vi "Main.vi"() -> ()   [LabVIEW 2013]
panel:
  in  "Upper Frequency Cutoff":dbl
  out "Derived Data":dbl[][](array[numeric])
  out "Processed Data":dbl[][](array[numeric])
  out "Raw Data":dbl[][](array[numeric])
  in  "Export Processed Data":bool
  in  "Process Data":bool
  in  "Time Units":enum16{"Seconds", "Minutes", "Hours"}(ring)
  in  "Data Type":enum16{"Raw", "Processed", "Derived"}(ring)
  in  "Derived Data to Display":enum16{"Altitude"}(ring)
  in  "Processed Data to Display":T1(ring)
  in  "Raw Data to Display":T1(ring)
  in  "Stop":bool
  out "error out":errorcluster
  in  "error in (no error)":errorcluster
  out "Displayed Data":cluster{dbl[], dbl[]}[](graph)
  in  "Raw Data File Path":path
  # "Processing Settings"
  # "Data Display Settings"
  # "Copyright (c) 2014 Andrew Donelick\nAll rights reserved. \n\nFor information, contact:\n<adonelick@hmc.edu>"
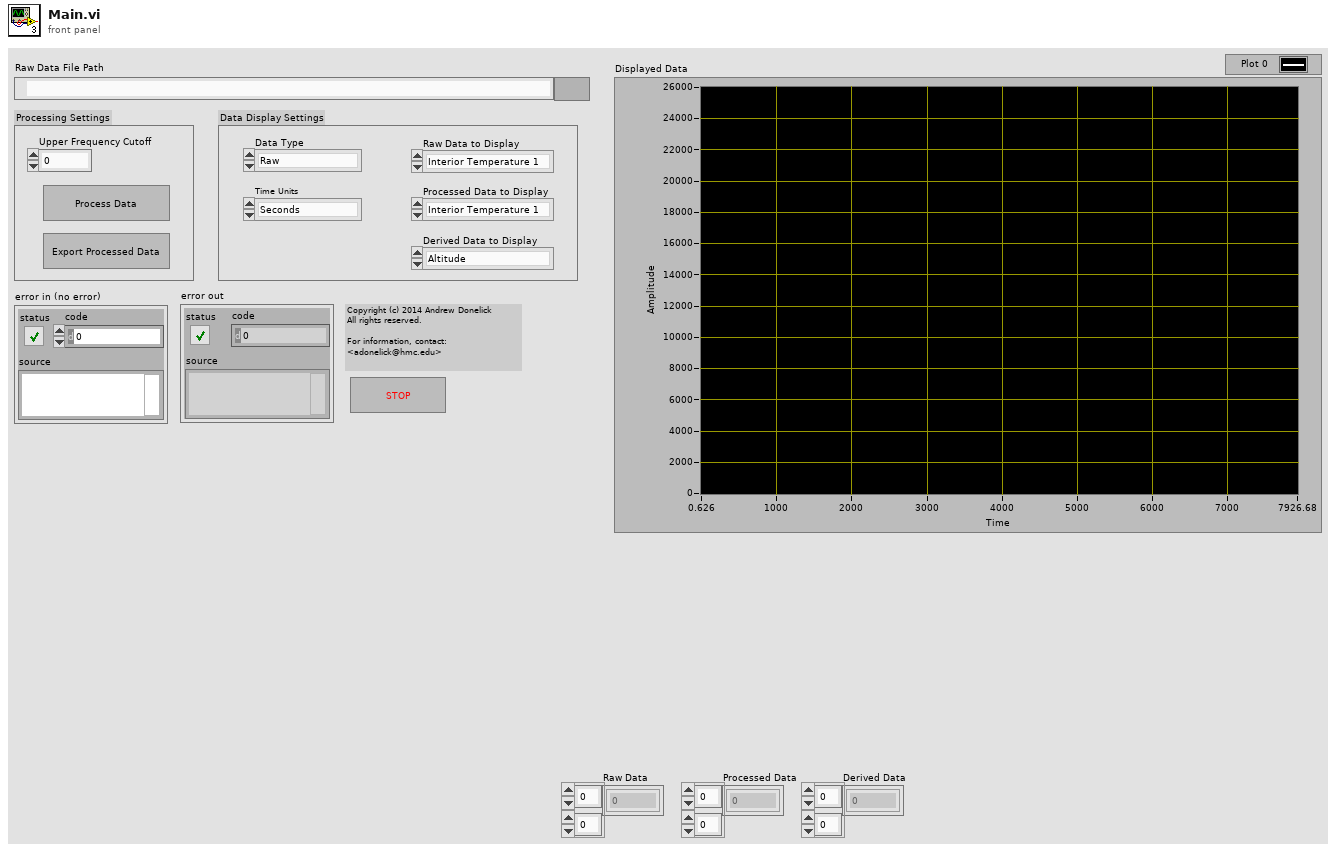
[diagram p1: front panel]
types:
  T1 = enum16{"Interior Temperature 1", "Interior Temperature 2", "Heater Temperature", "Exterior Temperature", "Humidity", "Pressure", "Pitch", "Roll", "Yaw", "Heater Status", "Relay States"}
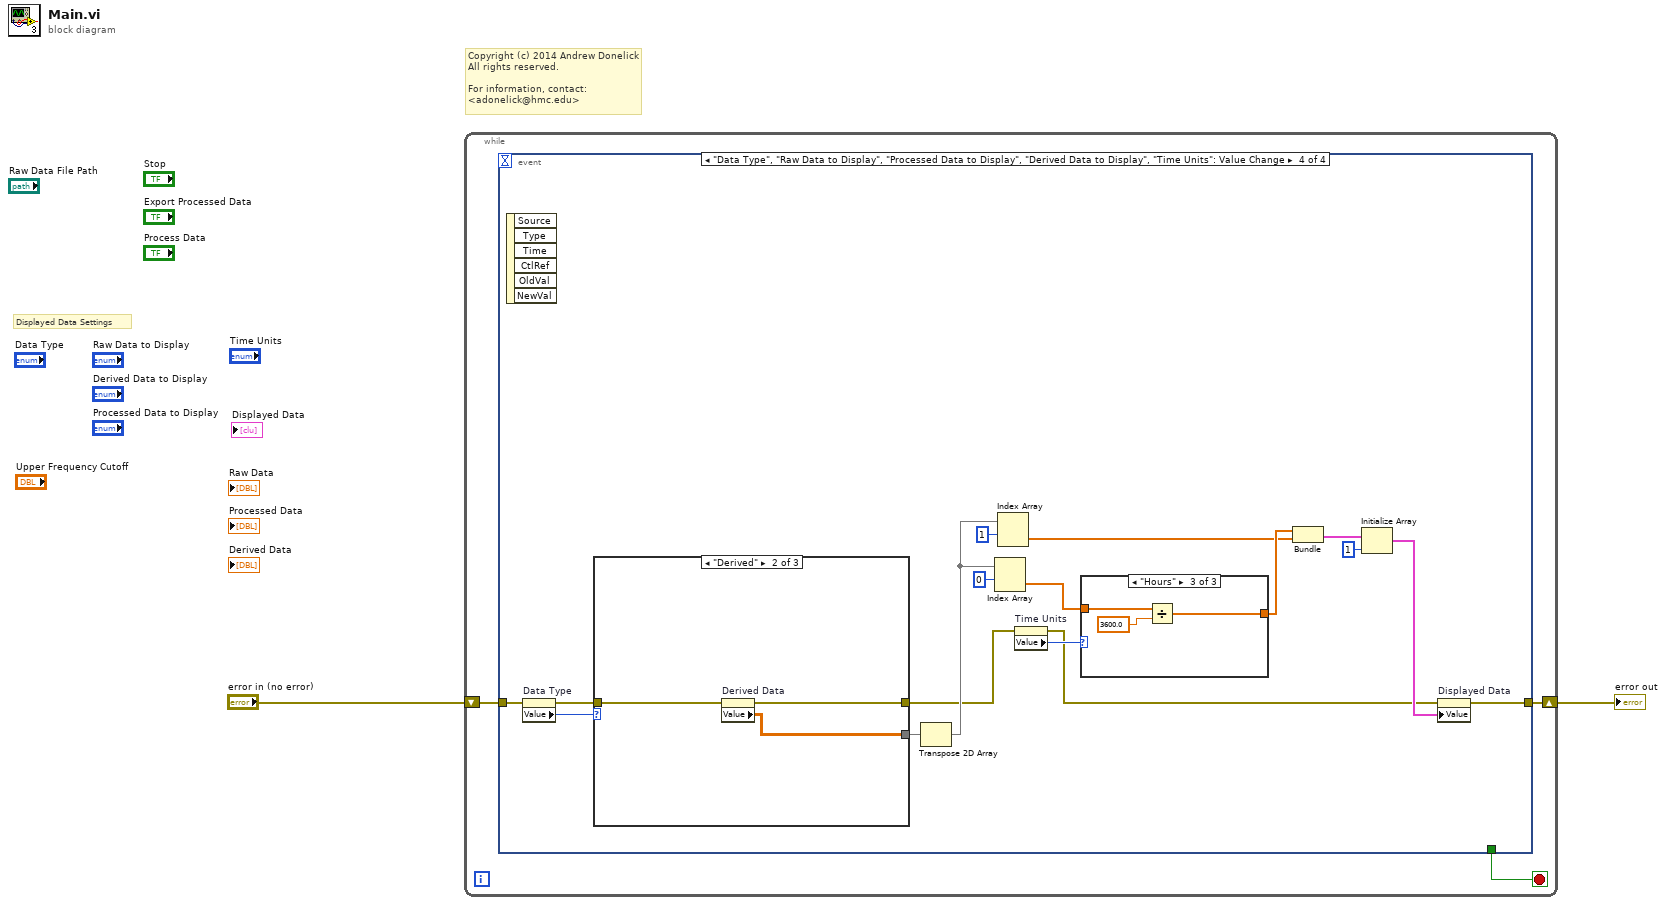
[diagram p0: block diagram]
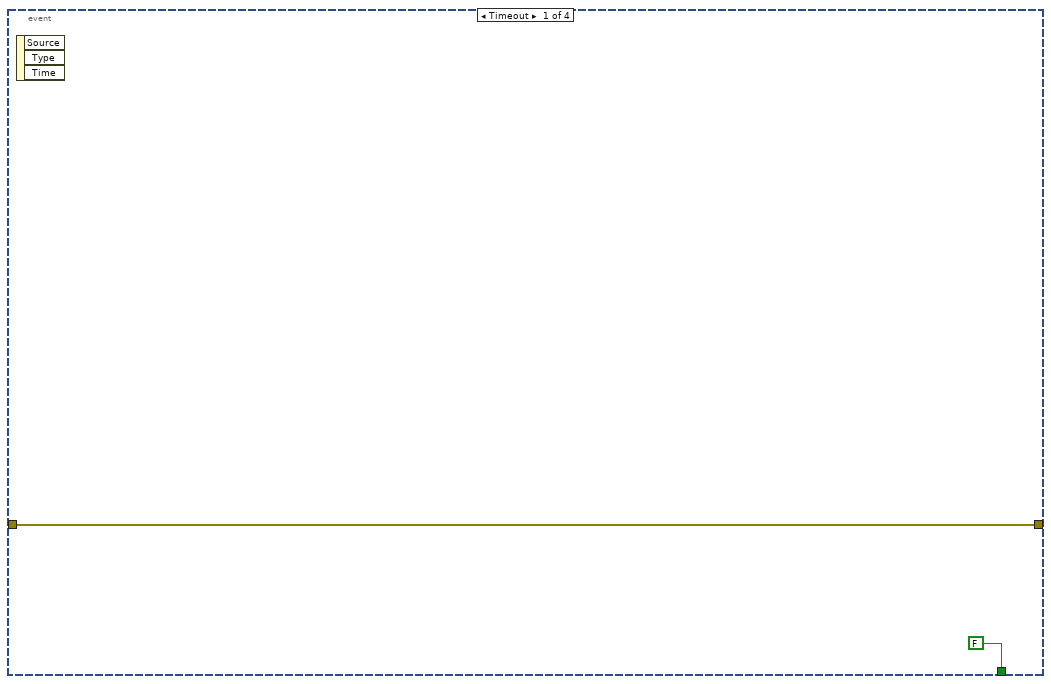
[diagram p2: hidden frame]
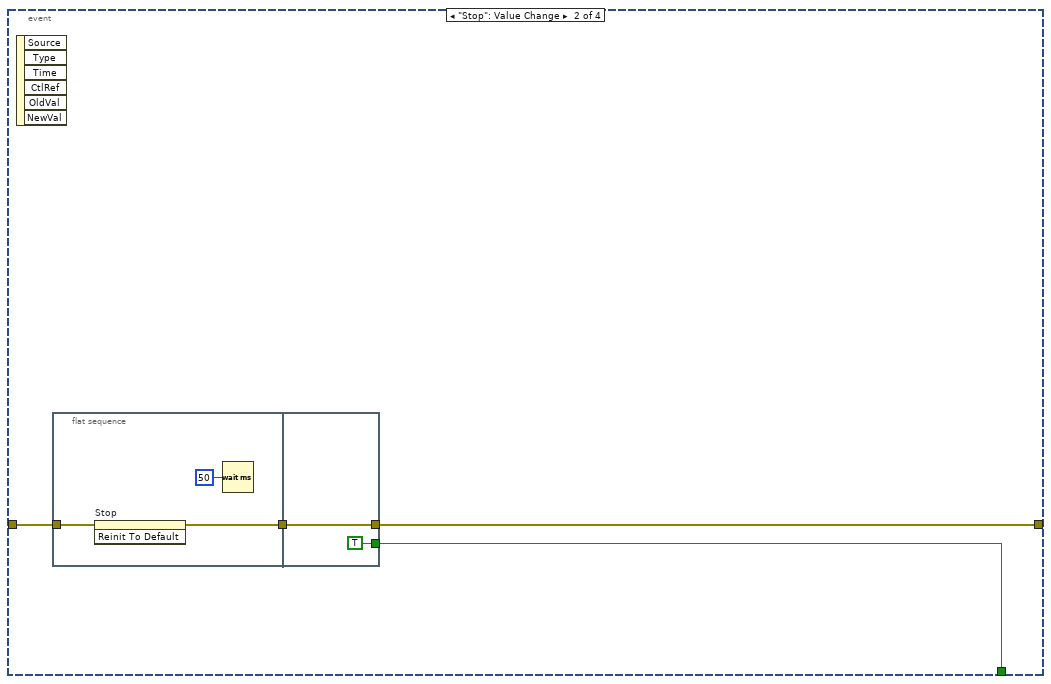
[diagram p3: hidden frame]
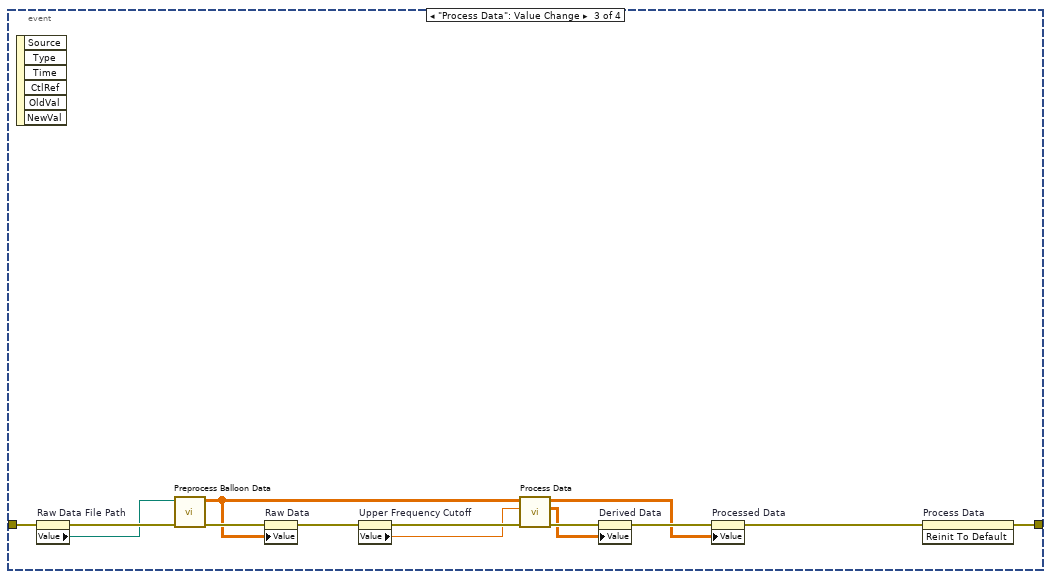
[diagram p4: hidden frame]
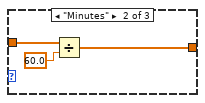
[diagram p6: hidden frame]
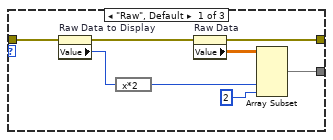
[diagram p7: hidden frame]
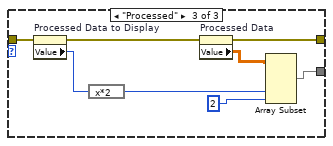
[diagram p8: hidden frame]
diagram:
  # "Copyright (c) 2014 Andrew Donelick\nAll rights reserved. \n\nFor information, contact:\n<adonelick@hmc.edu>"
  # "Displayed Data Settings"
  n1 = while {
    shift-right: [w3] -> w1
    shift-left: "error in (no error)" -> [w4]
    stop <- w5 stop-if-true
    n2 = event shown="[3] \"Data Type\", \"Raw Data to Display\", \"Processed Data to Display\", \"Derived Data to Display\", \"Time Units\": Value Change" {
      selector: _ -> [_ _ _ _]
      dyn-events: _ -> [_ _ _ _]
      timeout: _ -> [_ _ _ _]
      tunnel: [FALSE w9 _ _] -> w5
      tunnel: w4 -> [w6 w11 w29 w47]
      tunnel: [w6 w8 w30 w33] -> w3
      event Timeout {
        n3 = event-data() -> ()  [unwired: 1 in, 3 out]
      }
      event "Stop": Value Change {
        n4 = event-data() -> ()  [unwired: 1 in, 6 out]
        n5 = flat-sequence {
          tunnel: w11 -> [w14]
          tunnel: [w13] -> w10
          tunnel: w10 -> [w15]
          tunnel: [TRUE] -> w9
          tunnel: [w15] -> w8
          frame #0 {
            n6 = invoke on="Stop" class="Bool" method="Reinit To Default"(error in=w14) -> (error out=w13:errorcluster)  [unwired: 2 in, 2 out]
            n7 = Wait (ms)(milliseconds to wait=u32 50) -> ()  [unwired: 1 out]
          }
          frame #1 {
          }
        }
      }
      event "Process Data": Value Change {
        n8 = event-data() -> ()  [unwired: 1 in, 6 out]
        n9 = property on="Raw Data File Path" class="Path"(error in=w29) -> (error out=w28:errorcluster, "Value"=w27:path)  [unwired: 1 in, 1 out]
        n10 = call "Preprocess Balloon Data.vi"("error in (no error)"=w28, "Input Data File Path"=w27) -> ("error out"=w26:errorcluster, "Preprocessed Data"=w25:dbl[][])  [unwired: 8 in]
        n11 = property on="Raw Data" class="Arr (strict)"(error in=w26, "Value"=w25) -> (error out=w19:errorcluster)  [unwired: 1 in, 1 out]
        n12 = property on="Upper Frequency Cutoff" class="DigNum (strict)"(error in=w19) -> (error out=w18:errorcluster, "Value"=w17:dbl)  [unwired: 1 in, 1 out]
        n13 = call "Process Data.vi"("error in (no error)"=w18, "Upper Frequency Cutoff"=w17, "Raw Data"=w25) -> ("error out"=w24:errorcluster, "Altitude"=w22:dbl[][], "Processed Data"=w21:dbl[][])  [unwired: 6 in]
        n14 = property on="Derived Data" class="Arr (strict)"(error in=w24, "Value"=w22) -> (error out=w23:errorcluster)  [unwired: 1 in, 1 out]
        n15 = property on="Processed Data" class="Arr (strict)"(error in=w23, "Value"=w21) -> (error out=w20:errorcluster)  [unwired: 1 in, 1 out]
        n16 = invoke on="Process Data" class="Bool" method="Reinit To Default"(error in=w20) -> (error out=w30:errorcluster)  [unwired: 2 in, 2 out]
      }
      event "Data Type", "Raw Data to Display", "Processed Data to Display", "Derived Data to Display", "Time Units": Value Change {
        n17 = event-data() -> ()  [unwired: 1 in, 6 out]
        n18 = property on="Data Type" class="Enum (strict)"(error in=w47) -> (error out=w45:errorcluster, "Value"=w46:enum16{"Raw", "Processed", "Derived"})  [unwired: 1 in, 1 out]
        n19 = case shown="\"Derived\"" w46 {
          tunnel: w45 -> [w62 w65 w73]
          tunnel: [w55 w64 w72] -> w34
          tunnel: [w56 w63 w66] -> w35
          frame "Raw", Default {
            n20 = property on="Raw Data to Display" class="Enum (strict)"(error in=w62) -> (error out=w60:errorcluster, "Value"=w61:T1)  [unwired: 1 in, 1 out]
            n21 = expression code="x*2"(w61) -> (w58:T1)
            n22 = property on="Raw Data" class="Arr (strict)"(error in=w60) -> (error out=w55:errorcluster, "Value"=w59:dbl[][])  [unwired: 1 in, 1 out]
            n23 = Array Subset(array=w59, index (col)=w58, length (col)=2 ("length")) -> (w56:dbl[][])  [unwired: 2 in]
          }
          frame "Derived" {
            n24 = property on="Derived Data" class="Arr (strict)"(error in=w65) -> (error out=w64:errorcluster, "Value"=w63:dbl[][])  [unwired: 1 in, 1 out]
          }
          frame "Processed" {
            n25 = property on="Processed Data to Display" class="Enum (strict)"(error in=w73) -> (error out=w71:errorcluster, "Value"=w70:T1)  [unwired: 1 in, 1 out]
            n26 = expression code="x*2"(w70) -> (w68:T1)
            n27 = property on="Processed Data" class="Arr (strict)"(error in=w71) -> (error out=w72:errorcluster, "Value"=w69:dbl[][])  [unwired: 1 in, 1 out]
            n28 = Array Subset(array=w69, index (col)=w68, length (col)=2 ("disabled index (col)")) -> (w66:dbl[][])  [unwired: 2 in]
          }
        }
        n29 = Transpose 2D Array(2D array=w35) -> (transposed array=w41:dbl[][])
        n30 = Index Array(array=w41, index (row)=0) -> (element=w37:dbl[])  [unwired: 1 in]
        n31 = Index Array(array=w41, index (row)=1) -> (element=w31:dbl[])  [unwired: 1 in]
        n32 = property on="Time Units" class="Enum (strict)"(error in=w34) -> (error out=w36:errorcluster, "Value"=w38:enum16{"Seconds", "Minutes", "Hours"})  [unwired: 1 in, 1 out]
        n33 = case shown="\"Hours\"" w38 {
          tunnel: w37 -> [w48 w51 w54]
          tunnel: [w48 w49 w52] -> w32
          frame "Seconds", Default {
          }
          frame "Minutes" {
            n34 = Divide(x=w51, y=60.0) -> (x/y=w49:dbl[])
          }
          frame "Hours" {
            n35 = Divide(x=w54, y=3600.0) -> (x/y=w52:dbl[])
          }
        }
        n36 = Bundle(w32, w31) -> (w44:cluster{dbl[], dbl[]})  [unwired: 1 in]
        n37 = Initialize Array(w44, 1 ("dimension size")) -> (w42:cluster{dbl[], dbl[]}[])
        n38 = property on="Displayed Data" class="XYGraph (strict)"(error in=w36, "Value"=w42) -> (error out=w33:errorcluster)  [unwired: 1 in, 1 out]
      }
    }
  }
  "error out" <- w1
